vi "Transform2d_Equals.vi"(9 "otherTRANSFORM":T1={"TRANSLATION"={"X"=0.0, "Y"=0.0}, "ROTATION"={"VALUE"=0.0, "COS"=1.0, "SIN"=0.0}, "xF"=FALSE} {"ROTATION"."SIN" format="%13.4f"; "ROTATION"."COS" format="%13.4f"; "ROTATION"."VALUE" format="%13.4f"; "TRANSLATION"."Y" format="%14.3f"; "TRANSLATION"."X" format="%14.3f"}, 11 "inTRANSFORM":T1={"TRANSLATION"={"X"=0.0, "Y"=0.0}, "ROTATION"={"VALUE"=0.0, "COS"=1.0, "SIN"=0.0}, "xF"=FALSE} {"ROTATION"."SIN" format="%13.4f"; "ROTATION"."COS" format="%13.4f"; "ROTATION"."VALUE" format="%13.4f"; "TRANSLATION"."Y" format="%14.3f"; "TRANSLATION"."X" format="%14.3f"}) -> (3 "Equals":bool)   [LabVIEW 2019, in "Trajectory_Library.lvlib"]
doc: "Checks equality between this Transform2d and another object.\n\nParameters:\n - IN TRANSFORM - This TRANSFORM data structure\n - OTHER TRANSFORM - The other TRANSFORM to compare \n\nResults:\n - EQUALS - Returns TRUE when both TRANSFORMs are the same."
uses:
  Trajectory_Library.lvlib
  TypeDef/TRANSLATION2D.ctl
  TypeDef/ROTATION2D.ctl
  TypeDef/TRANSFORM2D.ctl
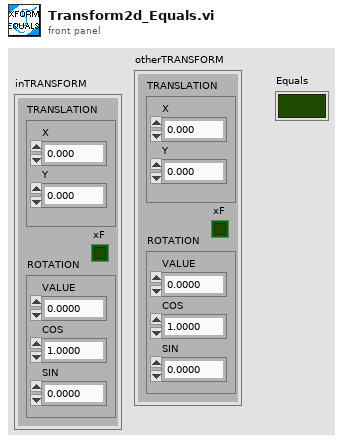
[diagram p1: front panel]
types:
  T1 = typedef "Trajectory_Library.lvlib/TRANSFORM2D.ctl" = cluster{"TRANSLATION":T2, "ROTATION":T3, "xF":bool}
  T2 = typedef "Trajectory_Library.lvlib/TRANSLATION2D.ctl" = cluster{"X":dbl, "Y":dbl}
  T3 = typedef "Trajectory_Library.lvlib/ROTATION2D.ctl" = cluster{"VALUE":dbl, "COS":dbl, "SIN":dbl}
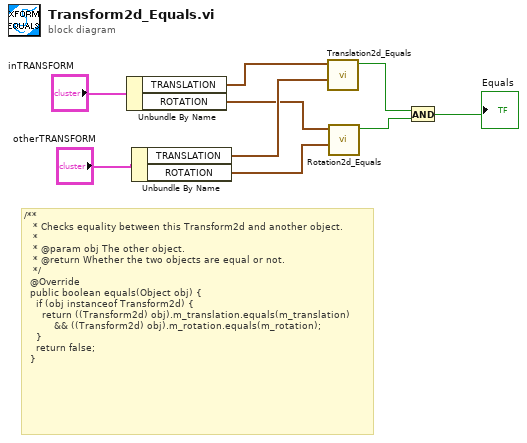
[diagram p0: block diagram]
diagram:
  # "/**\n   * Checks equality between this Transform2d and another object.\n   *\n   * @param obj The other object.\n   * @return Whether the two objects are equal or not.\n   */\n  @Override\n  public boolean equals(Object obj) {\n    if (obj instanceof Transform2d) {\n      return ((Transform2d) obj).m_translation.equals(m_translation)\n          && ((Transform2d) obj).m_rotation.equals(m_rotation);\n    }\n    return false;\n  }"
  n1 = Unbundle By Name("inTRANSFORM") -> ("TRANSLATION"=w7:T2, "ROTATION"=w5:T3)
  n2 = Unbundle By Name("otherTRANSFORM") -> ("TRANSLATION"=w6:T2, "ROTATION"=w4:T3)
  n3 = call "Translation2d_Equals.vi"("other Translation"=w6, "In Translation"=w7) -> ("Equals"=w3:bool)  [unwired: 9 in]
  n4 = call "Rotation2d_Equals.vi"("other ROTATION"=w4, "in ROTATION"=w5) -> ("Equals"=w2:bool)  [unwired: 9 in]
  n5 = And(x=w3, y=w2) -> (x .and. y?=→"Equals":bool)
